vi "Read Dev Margin.vi"(8 "error in (no error)":errorcluster, 11 "VISA resource name":refnum<visa-resource-name>) -> (0 "error out":errorcluster, 2 "dev margin":dbl, 3 "VISA resource name out":refnum<visa-resource-name>)   [LabVIEW 2021, in "Andeen-Hagerling 2700A.lvlib"]
doc: "Returns the value of the deviation mode margin parameter.\n\nThe deviation margin which controls the ability of the\nbridge to handle deviations outside of the input deviation\nbounds without encountering overloading of the preamplidier."
uses:
  Andeen-Hagerling 2700A.lvlib
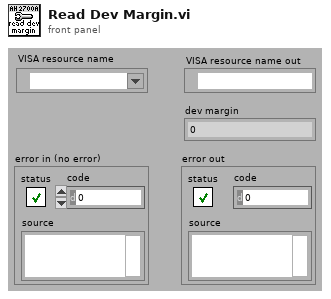
[diagram p1: front panel]
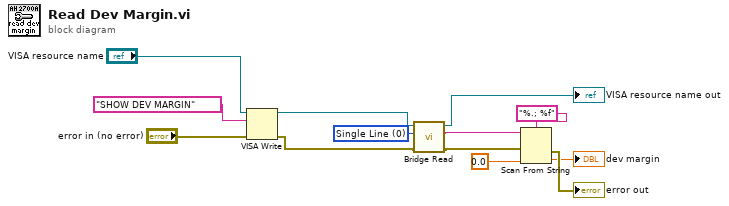
[diagram p0: block diagram]
diagram:
  w1 = u16 0 items=["Single Line", "Multi-Line"] ("Multiline")
  n1 = VISA Write(VISA resource name="VISA resource name", write buffer="SHOW DEV MARGIN" ("command"), error in (no error)="error in (no error)") -> (VISA resource name out=w6:refnum<visa-resource-name>, error out=w5:errorcluster)  [unwired: 1 out]
  n2 = call "Bridge Read.vi"("error in (no error)"=w5, "multiline"=w1, "VISA resource name"=w6) -> ("error out"=w4:errorcluster, "read buffer"=w3:string, "VISA resource name out"=→"VISA resource name out":refnum<visa-resource-name>)  [unwired: 6 in]
  n3 = Scan From String(format string="%.; %f", input string=w3, error in=w4, default 1=0.0 ("default value 1")) -> (error out=→"error out":errorcluster, output 1=→"dev margin":dbl)  [unwired: 1 in, 2 out]
